vi "NISE.remote.Get Property Access.vi"(0 "SLSC Remote in":refnum<class "SLSC Interface.lvclass">, 5 "property":refnum<k21>, 11 "error in (no error)":errorcluster) -> (4 "SLSC Remote out":refnum<class "SLSC Interface.lvclass">, 6 "property out":refnum<k21>, 10 "Prop.Access":i32(ring) items=["None", "Read Only", "Write Only", "Read/Write"], 15 "error out":errorcluster)   [LabVIEW 2016, in "SLSC Interface.lvclass"]
uses:
  SLSC Interface Class/SLSC Interface.lvclass
  SLSC Interface Class/SLSC Interface.lvclass/SLSC Interface.ctl
  SLSC Interface Class/NISE.Read client handle.vi
  SLSC Interface Class/NISE.Read URL.vi
  SLSC Interface Class/NISE.Read session.vi
  <vilib>/httpClient/POSTBuffer.vi
  <vilib>/NI/JSON Support for LabVIEW/JSON Value/Object/Get Value/Get Value (String).vi
  <vilib>/httpClient/LabVIEWHTTPClient.lvlib
  <vilib>/NI/JSON Support for LabVIEW/JSON Value/JSON Value.lvclass
  <vilib>/NI/NI JSONRPC Server Framework/Classes/Client/JSONRPC Client.lvclass
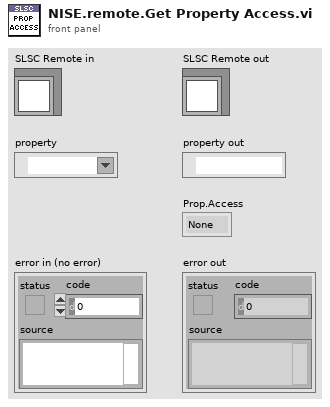
[diagram p1: front panel]
types:
  T1 = typedef "LabVIEWHTTPClient.lvlib/ClientHandle.ctl" = refnum<k1>
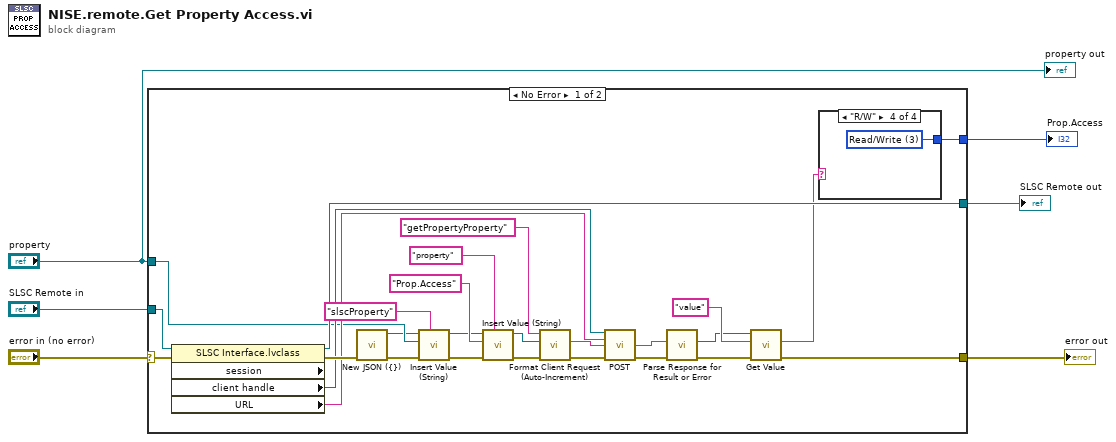
[diagram p0: block diagram]
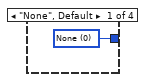
[diagram p2: hidden frame]
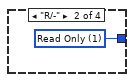
[diagram p3: hidden frame]
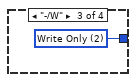
[diagram p4: hidden frame]
diagram:
  n1 = case shown="No Error" "error in (no error)" {
    selector: "error in (no error)" -> [w32 w39]
    tunnel: "SLSC Remote in" -> [w33 w38]
    tunnel: [w22 w39] -> w3
    tunnel: "property" -> [w11 _]
    tunnel: [w17 _] -> w4
    tunnel: [w16 w38] -> w1
    frame No Error {
      n2 = property class="SLSC Interface.lvclass" props=["session", "client handle", "URL"](reference=w33, error in=w32) -> (reference out=w16:refnum<class "SLSC Interface.lvclass">, error out=w31:errorcluster, "client handle"=w27:T1, "URL"=w26:string)  [unwired: 1 out]
      n3 = call <vilib>:"New JSON ({}).vi"("error in (no error)"=w31) -> ("error out"=w30:errorcluster, "JSON Value out"=w9:refnum<class "JSON Value.lvclass">)  [unwired: 9 in]
      n4 = call <vilib>:"Insert Value (String).vi"("key"="slscProperty" ("Name"), "error in (no error)"=w30, "value"=w11, "JSON Value in"=w9) -> ("error out"=w18:errorcluster, "JSON Value out"=w8:refnum<class "JSON Value.lvclass">)  [unwired: 5 in, 1 out]
      n5 = call <vilib>:"Insert Value (String).vi"("key"="property" ("Name"), "error in (no error)"=w18, "value"="Prop.Access" ("String"), "JSON Value in"=w8) -> ("error out"=w20:errorcluster, "JSON Value out"=w21:refnum<class "JSON Value.lvclass">)  [unwired: 5 in, 1 out]
      n6 = call <vilib>:"Format Client Request (Auto-Increment).vi"("error in (no error)"=w20, "JSON Value in"=w21, "method"="getPropertyProperty") -> ("error out"=w25:errorcluster, "Request String"=w28:string)  [unwired: 7 in]
      n7 = call-poly <vilib>:"POST.vi"("client handle"=w27, "url"=w26, "buffer"=w28, "error in (no error)"=w25) -> ("body"=w24:string, "error out"=w23:errorcluster)  [unwired: 8 in, 2 out]
      n8 = call <vilib>:"Parse Response for Result or Error.vi"("error in"=w23, "Response String In"=w24) -> ("error out"=w14:errorcluster, "JSON Value out"=w7:refnum<class "JSON Value.lvclass">)  [unwired: 7 in, 1 out]
      n9 = call-poly <vilib>:"Get Value.vi"("error in (no error)"=w14, "key"="value" ("Parameter Name"), "JSON Value in"=w7) -> ("error out"=w22:errorcluster, "value"=w15:string)  [unwired: 7 in]
      n10 = case shown="\"R/W\"" w15 {
        tunnel: [w34 w35 w36 w37] -> w17
        frame "None", Default {
          w34 = 0 items=["None", "Read Only", "Write Only", "Read/Write"] ("Prop.Access")
        }
        frame "R/-" {
          w35 = 1 items=["None", "Read Only", "Write Only", "Read/Write"] ("Prop.Access")
        }
        frame "-/W" {
          w36 = 2 items=["None", "Read Only", "Write Only", "Read/Write"] ("Prop.Access")
        }
        frame "R/W" {
          w37 = 3 items=["None", "Read Only", "Write Only", "Read/Write"] ("Prop.Access")
        }
      }
    }
    frame Error {
    }
  }
  "error out" <- w3
  "SLSC Remote out" <- w1
  "Prop.Access" <- w4
  "property out" <- "property"
